vi "Manipulator Query.vi"(8 "error in (no error)":errorcluster, 10 "Command":string, 11 "VISA resource in":refnum<visa-resource-name>="COM1") -> (0 "error out":errorcluster, 1 "Return count":u32, 2 "Response":string, 3 "VISA resource out":refnum<visa-resource-name>)   [LabVIEW 2012, in "Scientifica Manipulator Daemon.lvlib"]
uses:
  Scientifica Manipulator Daemon.lvlib
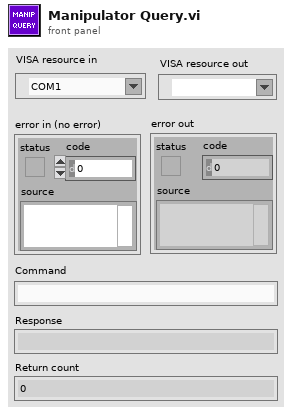
[diagram p1: front panel]
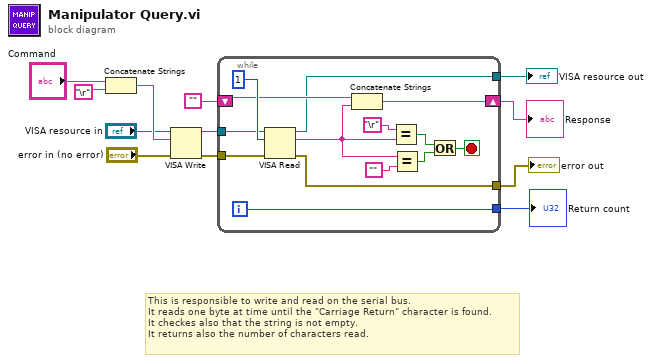
[diagram p0: block diagram]
diagram:
  # "This is responsible to write and read on the serial bus.\nIt reads one byte at time until the \"Carriage Return\" character is found.\nIt checkes also that the string is not empty.\nIt returns also the number of characters read."
  n1 = Concatenate Strings("Command", "\r") -> (w6:string)
  n2 = VISA Write(VISA resource name="VISA resource in", write buffer=w6, error in (no error)="error in (no error)") -> (VISA resource name out=w8:refnum<visa-resource-name>, error out=w9:errorcluster)  [unwired: 1 out]
  n3 = while {
    shift-right: [w25] -> w10
    shift-left: "" -> [w24]
    tunnel: [w23] -> w4
    tunnel: w9 -> [w22]
    tunnel: [w21] -> w3
    tunnel: w8 -> [w20]
    tunnel: [w19] -> w7
    i -> [w19]
    stop <- w13 stop-if-true
    n4 = VISA Read(VISA resource name=w20, byte count=u32 1, error in (no error)=w22) -> (VISA resource name out=w21:refnum<visa-resource-name>, read buffer=w18:string, error out=w23:errorcluster)  [unwired: 1 out]
    n5 = Concatenate Strings(w24, w18) -> (w25:string)
    n6 = Equal?(x="\r", y=w18) -> (x = y?=w14:bool)
    n7 = Equal?(x=w18, y="") -> (x = y?=w15:bool)
    n8 = Or(x=w14, y=w15) -> (x .or. y?=w13:bool)
  }
  "VISA resource out" <- w3
  "error out" <- w4
  "Response" <- w10
  "Return count" <- w7
